vi "Tooling Playground.vi"() -> ()   [LabVIEW 2019]
uses:
  Classes/Settings/Setting Database/Typedefs/PublicEvents--Setting Database.PathsUpdated.ctl
  Classes/Settings/Path Settings/Path Settings.lvclass
  Classes/Settings/Setting Database/Typedefs/PublicEvents--Setting Database.RectanglesUpdated.ctl
  Classes/Settings/Rectangle Settings/Rectangle Settings.lvclass
  C:/Users/Albro/Documents/GitHub/AFM-Lithography/lvsrc/Classes/Settings/ObjectSettings/ObjectSettings.lvclass
  Classes/Settings/Setting Database/Typedefs/PublicEvents--Setting Database.FunnelsUpdated.ctl
  Classes/Settings/Funnel Settings/Funnel Settings.lvclass
  Classes/Settings/Setting Database/Typedefs/PublicEvents--Setting Database.DotsUpdated.ctl
  Classes/Settings/Dot Settings/Dot Settings.lvclass
  Classes/Parse/ParsePaths/Path.lvclass
  Classes/Parse/Rectangle/Rectangle.lvclass
  Classes/Parse/Image/SVGImage.lvclass
  Classes/Parse/Dot/Dot.lvclass
  Classes/Parse/ParsePaths/Path.lvclass/Path.ctl
  Classes/Tool/Tool Rectangle/Tool Rectangle.lvclass
  Classes/Settings/ObjectSettings/ObjectSettings.lvclass/ObjectSettings.ctl
  Classes/Settings/Rectangle Settings/Rectangle Settings.lvclass/Rectangle Settings.ctl
  Classes/Tool/Tool Funnel/Tool Funnel.lvclass
  subVIs/typedefs/Schedule Types/Schedule--Formula.ctl
  Classes/Tool/Tool Path/Tool Path.lvclass
  Classes/Settings/Path Settings/Path Settings.lvclass/Path Settings.ctl
  Classes/Parse/PathCommands/PathCommands.lvclass
  Classes/Parse/Transform/Transform.lvclass
  Classes/Parse/PathCommands/Point.ctl
  Classes/Settings/ObjectSettings/ObjectSettings.lvclass
  Classes/Tool/Tool Object/Tool Object.lvclass
  Classes/Parse/PathCommands.Moveto/PathCommands.MoveTo.lvclass
  Classes/Parse/PathCommands.LineTo/PathCommands.LineTo.lvclass
  Classes/Parse/PathCommands.CurveTo/PathCommands.CurveTo.lvclass
  Classes/Parse/PathCommands.ClosePath/PathCommands.ClosePath.lvclass
  Classes/Parse/CSSProperties/CSSProperties.lvclass
  Classes/Parse/Transform.Translate/Transform.Translate.lvclass
  Classes/Parse/Transform.Matrix/Transform.Matrix.lvclass
  Classes/Settings/Setting Database/Setting Database.lvclass
panel:
  out "Object Sorting":u32
  out "Array":u32[](array[numeric])
  out "Numeric":i32
  out "Rect":u32
  out "Funnel":u32
  out "Path":u32
  in  "Fill Spacing":dbl=2.0 format="%#_13g"
  in  "Fill Orientation":u16(ring) items=["Horizontal", "Vertical"]
  out "XY Graph":cluster{dbl[], dbl[]}[](graph)
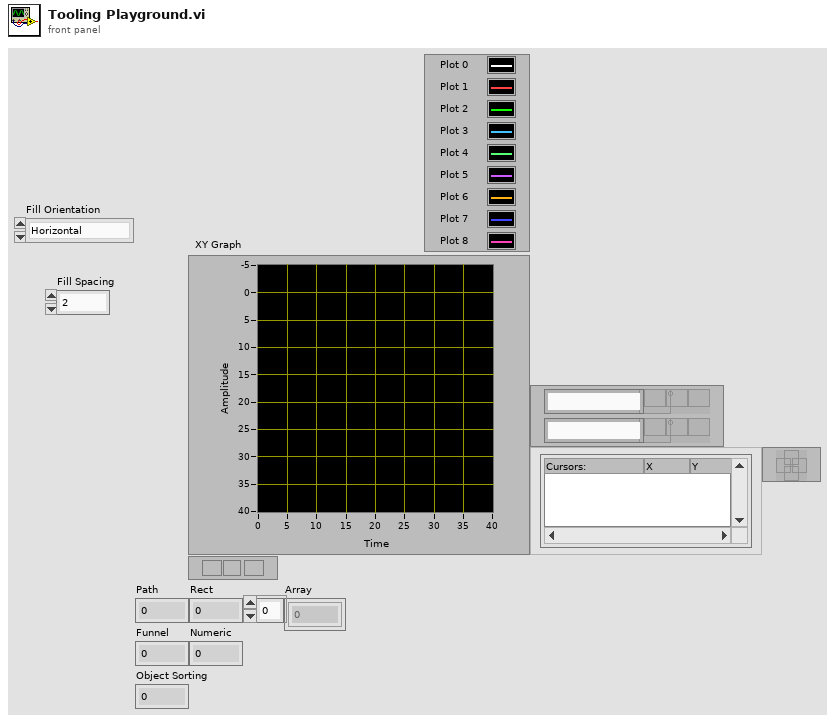
[diagram p1: front panel]
types:
  T1 = cluster{"Paths":refnum<class "Path.lvclass">[], "Rectangles":refnum<class "Rectangle.lvclass">[], "SVGImage":refnum<class "SVGImage.lvclass">, "Dots":refnum<class "Dot.lvclass">[]}
  T2 = typedef "Setting Database.lvclass/PublicEvents--Setting Database.PathsUpdated.ctl" = refnum<class "Path Settings.lvclass">[]
  T3 = typedef "Setting Database.lvclass/PublicEvents--Setting Database.RectanglesUpdated.ctl" = refnum<class "Rectangle Settings.lvclass">[]
  T4 = typedef "Setting Database.lvclass/PublicEvents--Setting Database.FunnelsUpdated.ctl" = refnum<class "Funnel Settings.lvclass">[]
  T5 = typedef "Setting Database.lvclass/PublicEvents--Setting Database.DotsUpdated.ctl" = refnum<class "Dot Settings.lvclass">[]
  T6 = cluster{"Paths":T2, "Rectangles":T3, "Funnels":T4, "Dots":T5}
  T7 = typedef "Schedule--Formula.ctl" = cluster{"formula":string, "formula length (nm)":dbl, "formula resolution (nm)":dbl}
  T8 = typedef "PathCommands.lvclass/Point.ctl" = cluster{"X":dbl, "Y":dbl}
  T9 = cluster{"Command Type":string, "Coordinates":cluster{"X":dbl, "Y":dbl}[]}[]
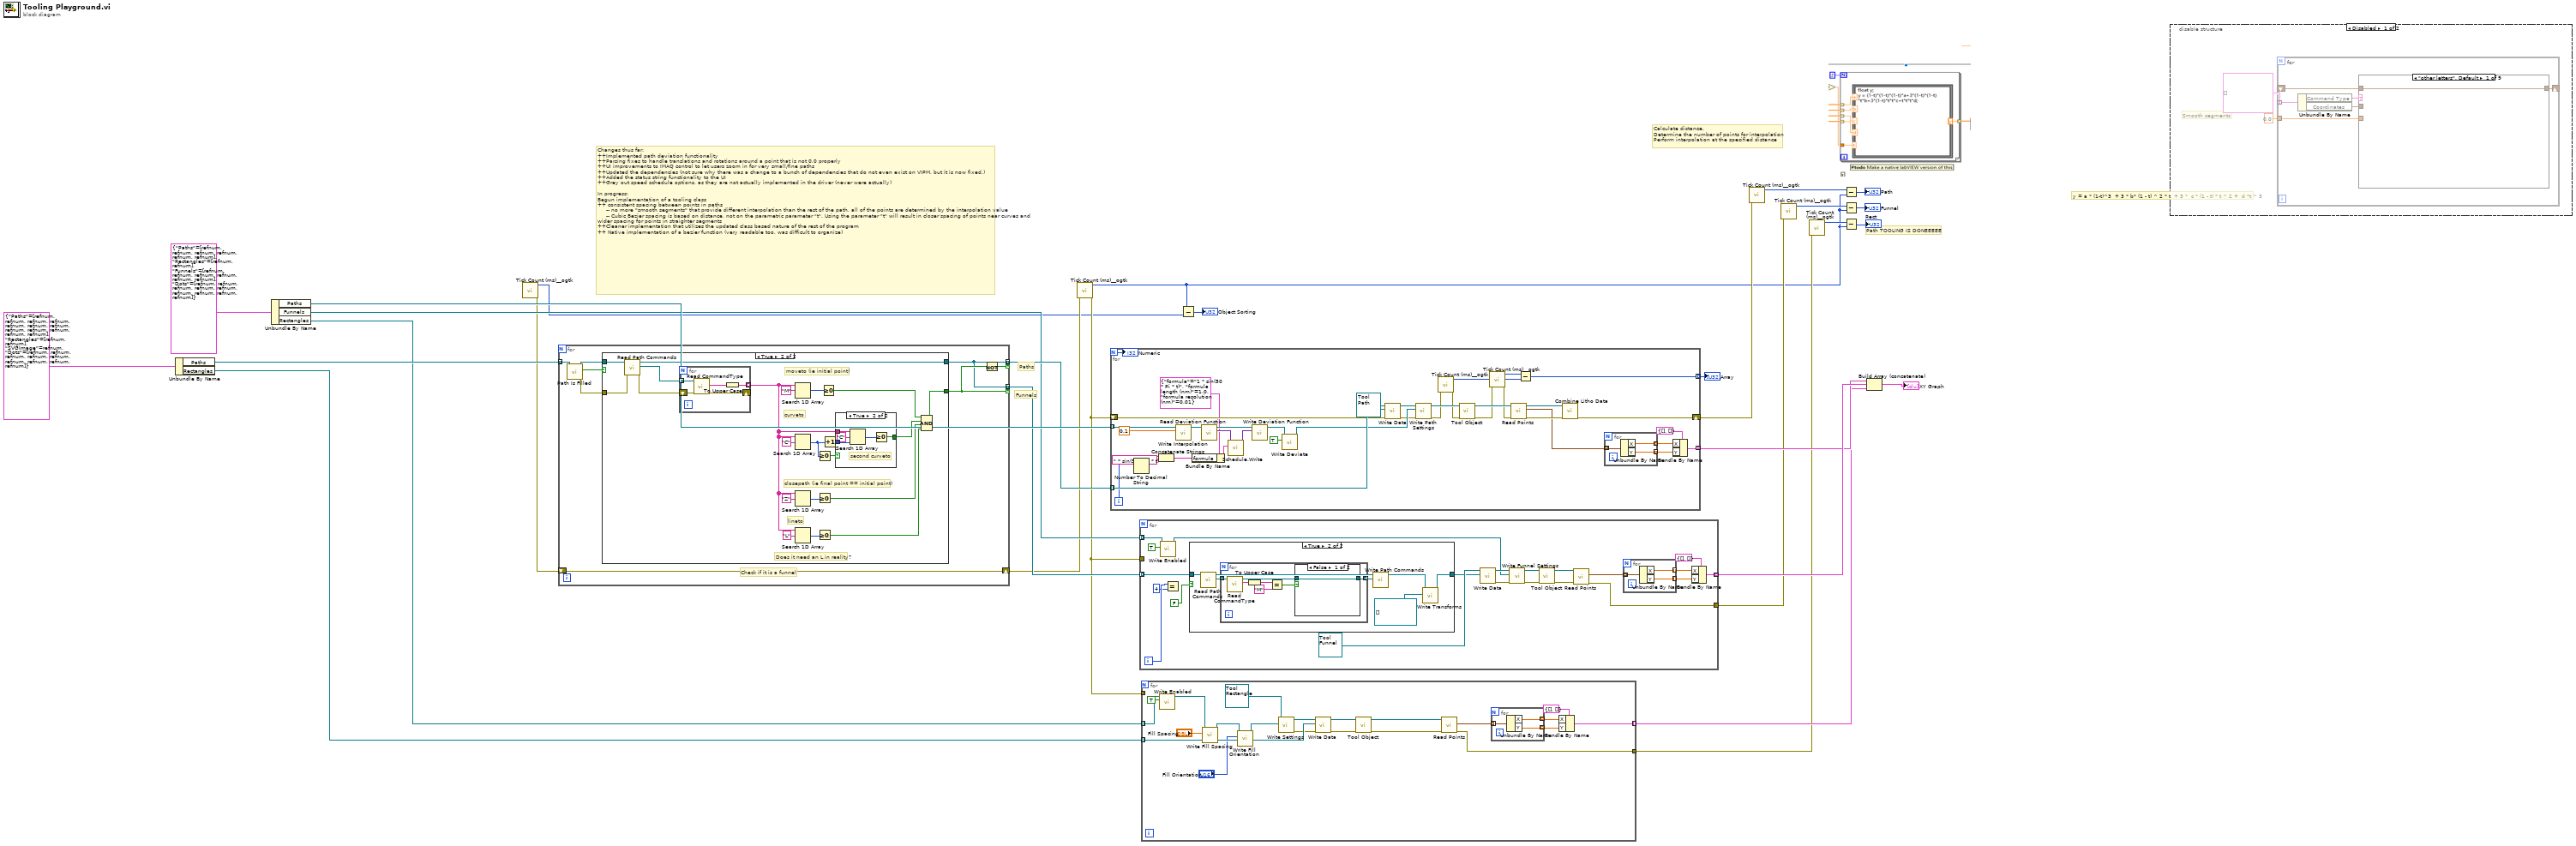
[diagram p0: block diagram]
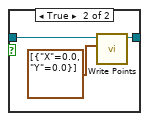
[diagram p3: hidden frame]
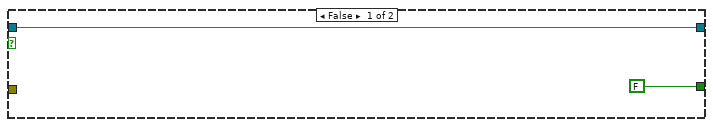
[diagram p4: hidden frame]
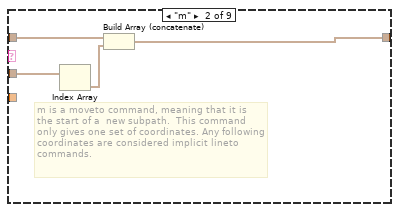
[diagram p6: hidden frame]
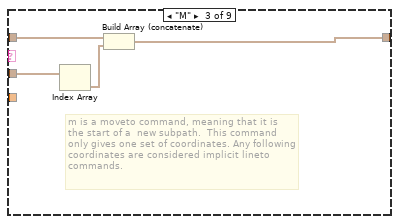
[diagram p7: hidden frame]
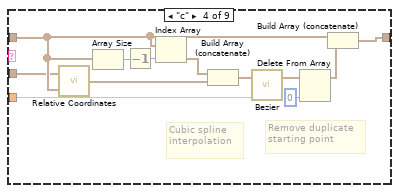
[diagram p8: hidden frame]
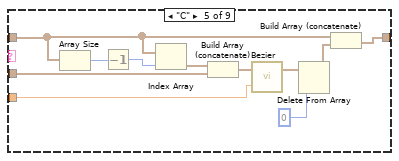
[diagram p9: hidden frame]
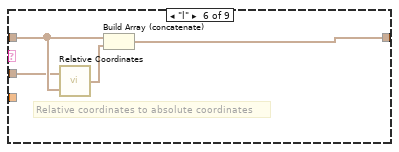
[diagram p10: hidden frame]
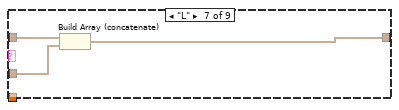
[diagram p11: hidden frame]
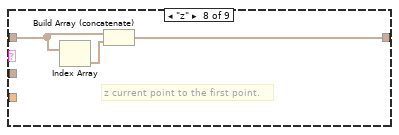
[diagram p12: hidden frame]
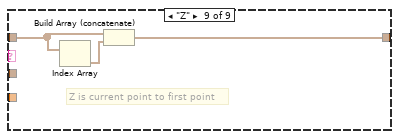
[diagram p13: hidden frame]
diagram:
  # "Changes thus far:\n++Implemented path deviation functionality\n++Parsing fixes to handle translations and rotations around a point that is not 0,0 properly\n++UI improvements to IMAQ control to let users zoom in for very small/fine paths\n++Updated the dependencies (not sure why there was a change to a bunch of dependencies that do not even exist on VIPM, but it is now fixed.)\n++Added the status string functionality to the UI\n++Grey out speed schedule options, as they are not actually implemented in the driver (never were actually)\n\nIn progress: \nBegun implementation of a tooling class\n++ consistent spacing between points in paths \n     -- no more \"smooth segments\" that provide different interpolation than the rest of the path, all of the points are determined by the interpolation value\n     -- Cubic Bezier spacing is based on distance, not on the parametric parameter \"t\". Using the parameter \"t\" will result in closer spacing of points near curves and wider spacing for points in straighter segments\n++Cleaner implementation that utilizes the updated class based nature of the rest of the program\n++ Native implementation of a bezier function (very readable too, was difficult to organize)"
  # "Path TOOLING IS DONEEEEE"
  # "Calculate distance.\nDetermine the number of points for interpolation\nPerform interpolation at the specified distance"
  # "y = a * (1-t)^3  + 3 * b* (1 - t) ^ 2 * t  + 3 *  c * (1 - t) * t ^ 2 +  d *t ^ 3"
  # "Funnels"
  # "Paths"
  n1 = Unbundle By Name(T1 {"Paths"=[refnum, refnum, refnum, refnum, refnum, refnum, refnum, refnum, refnum, refnum, refnum, refnum], "Rectangles"=[refnum, refnum], "SVGImage"=refnum, "Dots"=[refnum, refnum, refnum, refnum, refnum, refnum, refnum, refnum, refnum]}) -> ("Paths"=w29:refnum<class "Path.lvclass">[], "Rectangles"=w21:refnum<class "Rectangle.lvclass">[])
  n2 = Unbundle By Name(T6 {"Paths"=[refnum, refnum, refnum, refnum, refnum, refnum], "Rectangles"=[refnum, refnum], "Funnels"=[refnum, refnum, refnum, refnum, refnum, refnum], "Dots"=[refnum, refnum, refnum, refnum, refnum, refnum, refnum, refnum, refnum]} ("Response")) -> ("Paths"=w28:T2, "Funnels"=w25:T4, "Rectangles"=w20:T3)
  n3 = call <userlib>:"Tick Count (ms)__ogtk.vi"() -> ("error out"=w4:errorcluster, "millisecond timer value"=w2:u32)  [unwired: 10 in]
  n4 = for {
    tunnel: w29 -> [w31] mode=indexing
    tunnel: [w35] -> w27 mode=indexing if=w37
    tunnel: [w35] -> w26 mode=indexing if=w36
    shift-right: [w33] -> w5
    shift-left: w4 -> [w33]
    # "Check if it is a funnel"
    n5 = call "Path Is Filled.vi"("Path in"=w31) -> ("error out"=w30:errorcluster, "x != y?"=w34:bool, "Path out"=w32:refnum<class "Path.lvclass">)  [unwired: 8 in]
    n6 = case shown="True" w34 {
      tunnel: [FALSE w45] -> w36
      tunnel: w32 -> [w39 w44]
      tunnel: [w39 w43] -> w35
      tunnel: w30 -> [_ w40]
      frame False {
      }
      frame True {
        # "Does it need an L in reality?"
        # "lineto"
        # "closepath (ie final point == initial point)"
        # "curveto"
        # "moveto (ie initial point)"
        n7 = call "Read Path Commands.vi"("error in (no error)"=w40, "Path in"=w44) -> ("error out"=w41:errorcluster, "Path Commands"=w42:refnum<class "PathCommands.lvclass">[], "Path out"=w43:refnum<class "Path.lvclass">)  [unwired: 7 in]
        n8 = for {
          tunnel: w42 -> [w71] mode=indexing
          tunnel: [w69] -> w46 mode=indexing
          shift-right: [w67] -> _
          shift-left: w41 -> [w68]
          n9 = call-dynamic "Read CommandType.vi"("error in (no error)"=w68, "PathCommands in"=w71) -> ("error out"=w67:errorcluster, "CommandType"=w70:string)  [unwired: 7 in, 1 out]
          n10 = To Upper Case(1:w70) -> (0:w69:string)
        }
        n11 = Search 1D Array(1D array=w46, element="M") -> (index of element=w58:i32)  [unwired: 1 in]
        n12 = Search 1D Array(1D array=w46, element="C") -> (index of element=w57:i32)  [unwired: 1 in]
        n13 = Search 1D Array(1D array=w46, element="Z") -> (index of element=w54:i32)  [unwired: 1 in]
        n14 = Search 1D Array(1D array=w46, element="L") -> (index of element=w49:i32)  [unwired: 1 in]
        n15 = Greater Or Equal To 0?(x=w57) -> (x >= 0?=w56:bool)
        n16 = Greater Or Equal To 0?(x=w54) -> (x >= 0?=w51:bool)
        n17 = Greater Or Equal To 0?(x=w49) -> (x >= 0?=w47:bool)
        n18 = Greater Or Equal To 0?(x=w58) -> (x >= 0?=w53:bool)
        n19 = Increment(x=w57) -> (x+1=w50:i32)
        n20 = case shown="True" w56 {
          selector: w56 -> [w61 _]
          tunnel: w50 -> [_ w66]
          tunnel: w46 -> [_ w65]
          tunnel: [w61 w63] -> w52
          frame False {
          }
          frame True {
            # "second curveto"
            n21 = Search 1D Array(1D array=w65, element="C", start index (0)=w66) -> (index of element=w64:i32)
            n22 = Greater Or Equal To 0?(x=w64) -> (x >= 0?=w63:bool)
          }
        }
        n23 = Compound Arithmetic op=AND(w53, w52, w51, w47) -> (w45:bool)
      }
    }
    n24 = Not(x=w36) -> (.not. x?=w37:bool)
  }
  n25 = call <userlib>:"Tick Count (ms)__ogtk.vi"("error in (no error)"=w5) -> ("error out"=w16:errorcluster, "millisecond timer value"=w3:u32)  [unwired: 9 in]
  n26 = for {
    N -> [w85]
    tunnel: w28 -> [w107] mode=indexing
    tunnel: w27 -> [w109] mode=indexing
    shift-right: [w87] -> w15
    shift-left: w16 -> [w108]
    tunnel: [w89] -> w22 mode=indexing
    tunnel: [w78] -> w6 mode=indexing
    i -> [w75]
    n27 = Number To Decimal String(number=w75) -> (decimal integer string=w74:string)  [unwired: 1 in]
    n28 = Concatenate Strings(w74, " * sin(50 * Pi * t)" ("string")) -> (w72:string)
    n29 = call "Write Interpolation.vi"("Interpolation"=0.1, "Path Settings in"=w107) -> ("Path Settings out"=w102:refnum<class "Path Settings.lvclass">)  [unwired: 8 in, 1 out]
    n30 = Bundle By Name(cluster=T7 {"formula"="1 * sin(50 * Pi * t)", "formula length (nm)"=1.0, "formula resolution (nm)"=0.01} ("Formula"), "formula"=w72) -> (w76:T7)
    n31 = call-dynamic "Read Deviation Function.vi"("Path Settings in"=w102) -> ("Deviation Function"=w104:variant, "Path Settings out"=w105:refnum<class "Path Settings.lvclass">)  [unwired: 8 in, 1 out]
    n32 = call "Schedule.Write.vi"("Data to Write"=w76, "LUT In"=w104) -> ("LUT Out"=w103:variant)  [unwired: 8 in, 1 out]
    n33 = call-dynamic "Write Deviation Function.vi"("Deviation Function"=w103, "Path Settings in"=w105) -> ("Path Settings out"=w101:refnum<class "Path Settings.lvclass">)  [unwired: 8 in, 1 out]
    n34 = call-dynamic "Write Deviate.vi"("Deviate"=TRUE, "Path Settings in"=w101) -> ("Path Settings out"=w100:refnum<class "Path Settings.lvclass">)  [unwired: 8 in, 1 out]
    n35 = call-dynamic "Write Data.vi"("error in (no error)"=w108, "Path.lvclass"=w109, "Tool Path in"=refnum<class "Tool Path.lvclass"> refnum) -> ("error out"=w97:errorcluster, "Tool Path out"=w98:refnum<class "Tool Path.lvclass">)  [unwired: 7 in]
    n36 = call-dynamic "Write Path Settings.vi"("error in (no error)"=w97, "Path Settings.lvclass"=w100, "Tool Path in"=w98) -> ("error out"=w84:errorcluster, "Tool Path out"=w96:refnum<class "Tool Path.lvclass">)  [unwired: 7 in]
    n37 = call <userlib>:"Tick Count (ms)__ogtk.vi"("error in (no error)"=w84) -> ("error out"=w83:errorcluster, "millisecond timer value"=w79:u32)  [unwired: 9 in]
    n38 = call-dynamic "Tool Object.vi"("error in (no error)"=w83, "Tool Path in"=w96) -> ("error out"=w82:errorcluster, "Tool Path out"=w95:refnum<class "Tool Path.lvclass">)  [unwired: 8 in]
    n39 = call <userlib>:"Tick Count (ms)__ogtk.vi"("error in (no error)"=w82) -> ("error out"=w81:errorcluster, "millisecond timer value"=w80:u32)  [unwired: 9 in]
    n40 = call-dynamic "Read Points.vi"("error in (no error)"=w81, "Tool Object in"=w95) -> ("error out"=w93:errorcluster, "Points"=w88:T8[], "Tool Object out"=w94:refnum<class "Tool Path.lvclass">)  [unwired: 7 in]
    n41 = Subtract(x=w80, y=w79) -> (x-y=w78:u32)
    n42 = call-dynamic "Combine Litho Data.vi"("error in (no error)"=w93, "Tool Object in"=w94) -> ("error out"=w87:errorcluster)  [unwired: 7 in, 2 out]
    n43 = for {
      tunnel: w88 -> [w112] mode=indexing
      tunnel: [w111] -> w92 mode=indexing
      tunnel: [w110] -> w91 mode=indexing
      n44 = Unbundle By Name(w112) -> ("X"=w111:dbl, "Y"=w110:dbl)
    }
    n45 = Bundle By Name(cluster=cluster{"X":dbl[], "Y":dbl[]} {"X"=[], "Y"=[]} ("input cluster"), "X"=w92, "Y"=w91) -> (w89:cluster{"X":dbl[], "Y":dbl[]})
    "Numeric" <- w85
  }
  "Array" <- w6
  n46 = for {
    tunnel: w26 -> [w125] mode=indexing
    tunnel: w25 -> [w120] mode=indexing
    tunnel: [w114] -> w24 mode=indexing
    tunnel: w16 -> [_]
    tunnel: [w113] -> w14
    i -> [w124]
    n47 = call "Write Enabled.vi"("Enabled"=TRUE, "ObjectSettings in"=w120) -> ("ObjectSettings out"=w121:refnum<class "Funnel Settings.lvclass">)  [unwired: 8 in, 1 out]
    n48 = Equal?(x=w124, y=4) -> ()  [unwired: 1 out]
    n49 = case shown="True" FALSE {
      tunnel: [w137 w139] -> w126
      tunnel: w125 -> [w137 w144]
      frame False {
      }
      frame True {
        n50 = call "Read Path Commands.vi"("Path in"=w144) -> ("Path Commands"=w143:refnum<class "PathCommands.lvclass">[], "Path out"=w142:refnum<class "Path.lvclass">)  [unwired: 8 in, 1 out]
        n51 = for {
          tunnel: w143 -> [w151] mode=indexing
          tunnel: [w145] -> w141 mode=indexing
          n52 = call-dynamic "Read CommandType.vi"("PathCommands in"=w151) -> ("CommandType"=w150:string, "PathCommands out"=w146:refnum<class "PathCommands.lvclass">)  [unwired: 8 in, 1 out]
          n53 = To Upper Case(1:w150) -> (0:w149:string)
          n54 = Equal?(x=w149, y="M") -> (x = y?=w147:bool)
          n55 = case shown="False" w147 {
            tunnel: w146 -> [w152 w155]
            tunnel: [w152 w153] -> w145
            frame False {
            }
            frame True {
              n56 = call-dynamic "Write Points.vi"("Points"=T8[] [{"X"=0.0, "Y"=0.0}], "PathCommands in"=w155) -> ("PathCommands out"=w153:refnum<class "PathCommands.lvclass">)  [unwired: 8 in, 1 out]
            }
          }
        }
        n57 = call "Write Path Commands.vi"("Path Commands"=w141, "Path in"=w142) -> ("Path out"=w140:refnum<class "Path.lvclass">)  [unwired: 8 in, 1 out]
        n58 = call "Write Transforms.vi"("Transforms"=refnum<class "Transform.lvclass">[] [], "Path in"=w140) -> ("Path out"=w139:refnum<class "Path.lvclass">)  [unwired: 8 in, 1 out]
      }
    }
    n59 = call-dynamic "Write Data.vi"("Path.lvclass"=w126, "Tool Path in"=refnum<class "Tool Funnel.lvclass"> refnum ("Tool Funnel in")) -> ("error out"=w131:errorcluster, "Tool Path out"=w132:refnum<class "Tool Funnel.lvclass">)  [unwired: 8 in]
    n60 = call-dynamic "Write Funnel Settings.vi"("error in (no error)"=w131, "Funnel Settings.lvclass"=w121, "Tool Funnel in"=w132) -> ("error out"=w129:errorcluster, "Tool Funnel out"=w130:refnum<class "Tool Funnel.lvclass">)  [unwired: 7 in]
    n61 = call-dynamic "Tool Object.vi"("error in (no error)"=w129, "Tool Funnel in"=w130) -> ("error out"=w127:errorcluster, "Tool Funnel out"=w128:refnum<class "Tool Funnel.lvclass">)  [unwired: 8 in]
    n62 = call-dynamic "Read Points.vi"("error in (no error)"=w127, "Tool Object in"=w128) -> ("error out"=w113:errorcluster, "Points"=w118:T8[])  [unwired: 7 in, 1 out]
    n63 = for {
      tunnel: w118 -> [w136] mode=indexing
      tunnel: [w135] -> w117 mode=indexing
      tunnel: [w134] -> w116 mode=indexing
      n64 = Unbundle By Name(w136) -> ("X"=w135:dbl, "Y"=w134:dbl)
    }
    n65 = Bundle By Name(cluster=cluster{"X":dbl[], "Y":dbl[]} {"X"=[], "Y"=[]} ("input cluster"), "X"=w117, "Y"=w116) -> (w114:cluster{"X":dbl[], "Y":dbl[]})
  }
  n66 = for {
    tunnel: w21 -> [w174] mode=indexing
    tunnel: w20 -> [w169] mode=indexing
    tunnel: [w158] -> w19 mode=indexing
    tunnel: w16 -> [_]
    tunnel: [w156] -> w13
    n67 = call "Write Enabled.vi"("Enabled"=TRUE, "ObjectSettings in"=w169) -> ("ObjectSettings out"=w167:refnum<class "Rectangle Settings.lvclass">)  [unwired: 8 in, 1 out]
    n68 = call "Write Fill Spacing.vi"("Fill Spacing"="Fill Spacing", "Rectangle Settings in"=w167) -> ("Rectangle Settings out"=w165:refnum<class "Rectangle Settings.lvclass">)  [unwired: 8 in, 1 out]
    n69 = call "Write Fill Orientation.vi"("Fill Orientation"="Fill Orientation", "Rectangle Settings in"=w165) -> ("Rectangle Settings out"=w164:refnum<class "Rectangle Settings.lvclass">)  [unwired: 8 in, 1 out]
    n70 = call-dynamic "Write Settings.vi"("Rectangle Settings.lvclass"=w164, "Tool Rectangle in"=refnum<class "Tool Rectangle.lvclass"> refnum) -> ("error out"=w173:errorcluster, "Tool Rectangle out"=w175:refnum<class "Tool Rectangle.lvclass">)  [unwired: 8 in]
    n71 = call-dynamic "Write Data.vi"("error in (no error)"=w173, "Rectangle.lvclass"=w174, "Tool Rectangle in"=w175) -> ("error out"=w171:errorcluster, "Tool Rectangle out"=w172:refnum<class "Tool Rectangle.lvclass">)  [unwired: 7 in]
    n72 = call-dynamic "Tool Object.vi"("error in (no error)"=w171, "Tool Rectangle in"=w172) -> ("error out"=w157:errorcluster, "Tool Rectangle out"=w168:refnum<class "Tool Rectangle.lvclass">)  [unwired: 8 in]
    n73 = call-dynamic "Read Points.vi"("error in (no error)"=w157, "Tool Object in"=w168) -> ("error out"=w156:errorcluster, "Points"=w159:T8[])  [unwired: 7 in, 1 out]
    n74 = for {
      tunnel: w159 -> [w179] mode=indexing
      tunnel: [w178] -> w162 mode=indexing
      tunnel: [w177] -> w161 mode=indexing
      n75 = Unbundle By Name(w179) -> ("X"=w178:dbl, "Y"=w177:dbl)
    }
    n76 = Bundle By Name(cluster=cluster{"X":dbl[], "Y":dbl[]} {"X"=[], "Y"=[]} ("input cluster"), "X"=w162, "Y"=w161) -> (w158:cluster{"X":dbl[], "Y":dbl[]})
  }
  n77 = Subtract(x=w3, y=w2) -> (x-y=→"Object Sorting":u32)
  n78 = call <userlib>:"Tick Count (ms)__ogtk.vi"("error in (no error)"=w15) -> ("millisecond timer value"=w12:u32)  [unwired: 9 in, 1 out]
  n79 = call <userlib>:"Tick Count (ms)__ogtk.vi"("error in (no error)"=w14) -> ("millisecond timer value"=w11:u32)  [unwired: 9 in, 1 out]
  n80 = call <userlib>:"Tick Count (ms)__ogtk.vi"("error in (no error)"=w13) -> ("millisecond timer value"=w10:u32)  [unwired: 9 in, 1 out]
  n81 = Subtract(x=w12, y=w3) -> (x-y=→"Path":u32)
  n82 = Subtract(x=w11, y=w3) -> (x-y=→"Funnel":u32)
  n83 = Subtract(x=w10, y=w3) -> (x-y=→"Rect":u32)
  n84 = Build Array (concatenate)(w22, w24, w19) -> (→"XY Graph":cluster{"X":dbl[], "Y":dbl[]}[])
  n85 = disable-structure shown="Disabled" {
    frame Disabled {
      # "Smooth segments"
      n86 = for {
        tunnel: T9 [] ("Commands") -> [w187] mode=indexing
        shift-right: [w183] -> _
        shift-left: _ -> [w184]
        tunnel: 0.0 ("Smooth Segments") -> [w182]
        n87 = Unbundle By Name(w187) -> ("Command Type"=w186:string, "Coordinates"=w185:cluster{"X":dbl, "Y":dbl}[])
        n88 = case shown="\"other letters\", Default" w186 {
          tunnel: w185 -> [_ w192 w194 w201 w212 w220 w224 _ _]
          tunnel: w184 -> [w188 w191 w195 w207 w218 w222 w226 w228 w232]
          tunnel: [w188 w189 w193 w208 w219 w221 w225 w227 w230] -> w183
          tunnel: w182 -> [_ _ _ w200 w213 _ _ _ _]
          frame "other letters", Default {
          }
          frame "m" {
            # "m is a moveto command, meaning that it is the start of a  new subpath.  This command only gives one set of coordinates. Any following coordinates are considered implicit lineto commands."
            n89 = Index Array(array=w192) -> (element=w190:cluster{"X":dbl, "Y":dbl})  [unwired: 1 in]
            n90 = Build Array (concatenate)(w191, w190) -> (w189:cluster{"X":dbl, "Y":dbl}[])
          }
          frame "M" {
            # "m is a moveto command, meaning that it is the start of a  new subpath.  This command only gives one set of coordinates. Any following coordinates are considered implicit lineto commands."
            n91 = Index Array(array=w194) -> (element=w196:cluster{"X":dbl, "Y":dbl})  [unwired: 1 in]
            n92 = Build Array (concatenate)(w195, w196) -> (w193:cluster{"X":dbl, "Y":dbl}[])
          }
          frame "c" {
            # "Remove duplicate starting point"
            # "Cubic spline interpolation"
            n93 = call "Relative Coordinates.vi"("All Coordinates"=w207, "Command Coordinates"=w201) -> ("Adjusted Command Coordinates"=w205:cluster{"X":dbl, "Y":dbl}[])
            n94 = Array Size(array=w207) -> (size(s)=w203:i32)
            n95 = Decrement(x=w203) -> (x-1=w202:i32)
            n96 = Index Array(array=w207, index=w202) -> (element=w206:cluster{"X":dbl, "Y":dbl})
            n97 = Build Array (concatenate)(w206, w205) -> (w204:cluster{"X":dbl, "Y":dbl}[])
            n98 = call "Bezier.vi"("Segments"=w200, "Parameters"=w204) -> ("Coordinate Array"=w199:cluster{"X":dbl, "Y":dbl}[])  [unwired: 1 out]
            n99 = Delete From Array(array=w199, index=0) -> (array with subset deleted=w198:cluster{"X":dbl, "Y":dbl}[])  [unwired: 1 in, 1 out]
            n100 = Build Array (concatenate)(w207, w198) -> (w208:cluster{"X":dbl, "Y":dbl}[])
          }
          frame "C" {
            n101 = Array Size(array=w218) -> (size(s)=w215:i32)
            n102 = Decrement(x=w215) -> (x-1=w214:i32)
            n103 = Index Array(array=w218, index=w214) -> (element=w217:cluster{"X":dbl, "Y":dbl})
            n104 = Build Array (concatenate)(w217, w212) -> (w216:cluster{"X":dbl, "Y":dbl}[])
            n105 = call "Bezier.vi"("Segments"=w213, "Parameters"=w216) -> ("Coordinate Array"=w211:cluster{"X":dbl, "Y":dbl}[])  [unwired: 1 out]
            n106 = Delete From Array(array=w211, index=0) -> (array with subset deleted=w210:cluster{"X":dbl, "Y":dbl}[])  [unwired: 1 in, 1 out]
            n107 = Build Array (concatenate)(w218, w210) -> (w219:cluster{"X":dbl, "Y":dbl}[])
          }
          frame "l" {
            # "Relative coordinates to absolute coordinates"
            n108 = call "Relative Coordinates.vi"("All Coordinates"=w222, "Command Coordinates"=w220) -> ("Adjusted Command Coordinates"=w223:cluster{"X":dbl, "Y":dbl}[])
            n109 = Build Array (concatenate)(w222, w223) -> (w221:cluster{"X":dbl, "Y":dbl}[])
          }
          frame "L" {
            n110 = Build Array (concatenate)(w226, w224) -> (w225:cluster{"X":dbl, "Y":dbl}[])
          }
          frame "z" {
            # "z current point to the first point."
            n111 = Index Array(array=w228) -> (element=w229:cluster{"X":dbl, "Y":dbl})  [unwired: 1 in]
            n112 = Build Array (concatenate)(w228, w229) -> (w227:cluster{"X":dbl, "Y":dbl}[])
          }
          frame "Z" {
            # "Z is current point to first point"
            n113 = Index Array(array=w232) -> (element=w231:cluster{"X":dbl, "Y":dbl})  [unwired: 1 in]
            n114 = Build Array (concatenate)(w232, w231) -> (w230:cluster{"X":dbl, "Y":dbl}[])
          }
        }
      }
    }
    frame Enabled {
    }
  }
